vi "VALVE_change_2_way_valve_position.vi"(3 "error in":errorcluster, 4 "Valve position":bool, 5 "VISA valve":refnum<visa-resource-name>) -> (0 "error out":errorcluster, 2 "Valve error":bool)   [LabVIEW 2015]
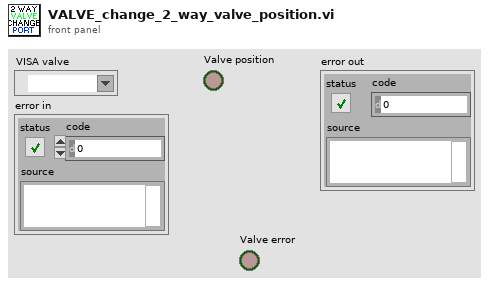
[diagram p1: front panel]
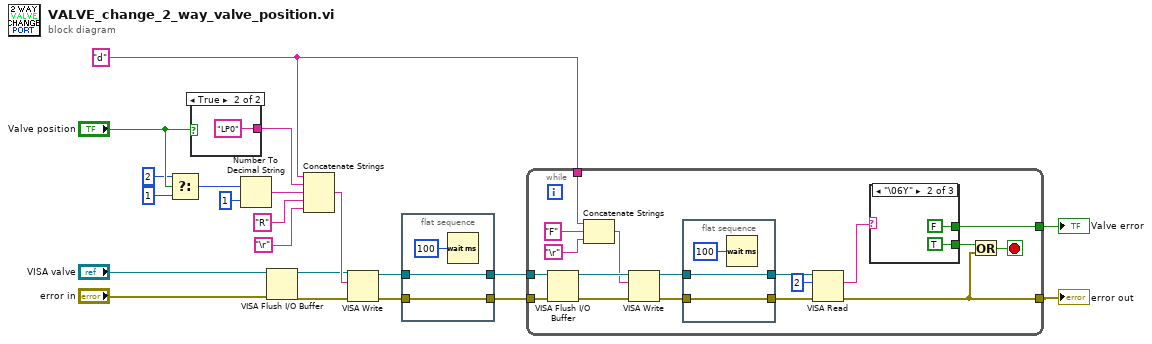
[diagram p0: block diagram]
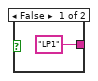
[diagram p2: hidden frame]
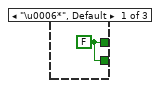
[diagram p3: hidden frame]
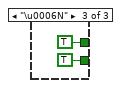
[diagram p4: hidden frame]
diagram:
  w7 = "d"
  n1 = Select(t=i16 2, s="Valve position", f=i16 1) -> (s? t:f=w2:i16)
  n2 = case shown="True" "Valve position" {
    tunnel: ["LP1" ("buffer d'écriture") "LP0" ("buffer d'écriture")] -> w8
    frame False {
    }
    frame True {
    }
  }
  n3 = Number To Decimal String(number=w2, width (-)=i16 1) -> (decimal integer string=w17:string)
  n4 = VISA Flush I/O Buffer(VISA resource name="VISA valve", error in (no error)="error in") -> (VISA resource name out=w13:refnum<visa-resource-name>, error out=w14:errorcluster)  [unwired: 1 in]
  n5 = Concatenate Strings(w7, w8, w17, "R" ("string"), "\r") -> (w16:string)
  n6 = VISA Write(VISA resource name=w13, write buffer=w16, error in (no error)=w14) -> (VISA resource name out=w12:refnum<visa-resource-name>, error out=w10:errorcluster)  [unwired: 1 out]
  n7 = flat-sequence {
    tunnel: w12 -> [w26]
    tunnel: [w26] -> w11
    tunnel: w10 -> [w25]
    tunnel: [w25] -> w9
    frame #0 {
      n8 = Wait (ms)(milliseconds to wait=u32 100) -> ()  [unwired: 1 out]
    }
  }
  n9 = while {
    tunnel: w9 -> [w38]
    tunnel: w11 -> [w37]
    tunnel: [w28] -> w1
    tunnel: w7 -> [w31]
    tunnel: [w27] -> w6
    stop <- w30 stop-if-true
    n10 = VISA Flush I/O Buffer(VISA resource name=w37, error in (no error)=w38) -> (VISA resource name out=w36:refnum<visa-resource-name>, error out=w35:errorcluster)  [unwired: 1 in]
    n11 = Concatenate Strings(w31, "F" ("string"), "\r") -> (w33:string)
    n12 = VISA Write(VISA resource name=w36, write buffer=w33, error in (no error)=w35) -> (VISA resource name out=w40:refnum<visa-resource-name>, error out=w41:errorcluster)  [unwired: 1 out]
    n13 = flat-sequence {
      tunnel: w40 -> [w52]
      tunnel: [w52] -> w42
      tunnel: w41 -> [w51]
      tunnel: [w51] -> w43
      frame #0 {
        n14 = Wait (ms)(milliseconds to wait=u32 100) -> ()  [unwired: 1 out]
      }
    }
    n15 = VISA Read(VISA resource name=w42, byte count=u32 2, error in (no error)=w43) -> (read buffer=w32:string, error out=w28:errorcluster)  [unwired: 2 out]
    n16 = case shown="\"\\06Y\"" w32 {
      tunnel: [w45 FALSE TRUE] -> w27
      tunnel: [w45 TRUE TRUE] -> w29
      frame "\u0006*", Default {
        w45 = FALSE
      }
      frame "\u0006Y" {
      }
      frame "\u0006N" {
      }
    }
    n17 = Or(x=w29, y=w28) -> (x .or. y?=w30:bool)
  }
  "error out" <- w1
  "Valve error" <- w6
